vi "Framework Configuration 1.0 JSON Flatten.vi"(8 "error in (no error)":errorcluster, 11 "framework configuration 1.0":T2) -> (0 "error out":errorcluster, 2 "dsf version":T1, 3 "dsf configuration json":string)   [LabVIEW 2017, in "DSF Core.lvlib" / "Configuration Session.lvclass"]
uses:
  Configuration Session.lvclass
  Typedefs/DSF Version Info.ctl
  DSF Core.lvlib
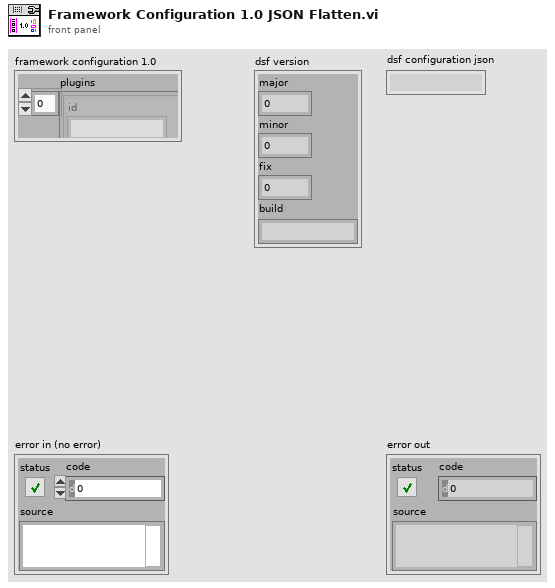
[diagram p1: front panel]
types:
  T1 = typedef "DSF Core.lvlib/DSF Version Info.ctl" = cluster{"major":u32, "minor":u32, "fix":u32, "build":string}
  T2 = cluster{"plugins":cluster{"id":string, "values":cluster{"components":string[], "timing":cluster{"priority":u64, "decimation":u64, "offset":u64}, "group ids":string[], "settings id":string, "threads":cluster{"buffer converter settings":cluster{"key":string, "value":string}[], "transceiver settings":cluster{"key":string, "value":string}[], "custom settings":cluster{"key":string, "value":string}[], "processor":i32, "priority offset":i16}[]}}[], "groups":cluster{"id":string, "values":cluster{"direction":i32, "timing":cluster{"priority":u64, "decimation":u64, "offset":u64}, "transfer ids":string[], "settings id":string, "thread":i32, "timeout behavior":u8}}[], "transfers":cluster{"id":string, "values":cluster{"byte order":i32, "channel ids":string[], "settings id":string}}[], "channels":cluster{"id":string, "values":cluster{"string buffer offset":u64, "string data type":i32, "engine data type":i32, "settings id":string, "units":string}}[], "settings":cluster{"id":string, "values":cluster{"key":string, "value":string}[]}[]}
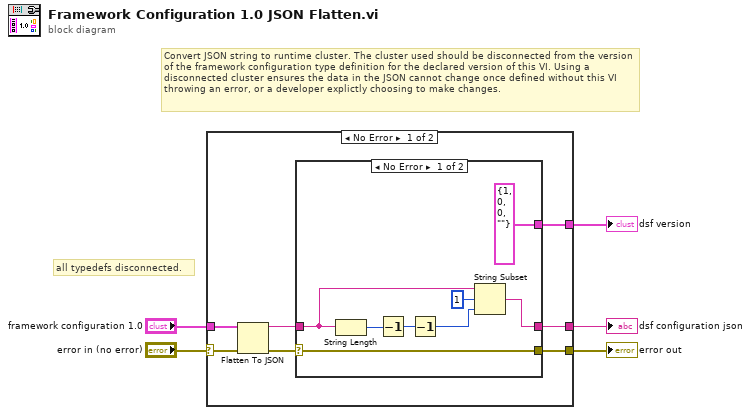
[diagram p0: block diagram]
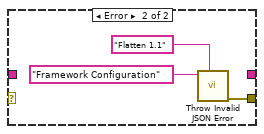
[diagram p2: hidden frame]
diagram:
  # "all typedefs disconnected."
  # "Convert JSON string to runtime cluster. The cluster used should be disconnected from the version of the framework configuration type definition for the declared version of this VI. Using a disconnected cluster ensures the data in the JSON cannot change once defined without this VI throwing an error, or a developer explictly choosing to make changes."
  n1 = case shown="No Error" "error in (no error)" {
    selector: "error in (no error)" -> [w9 w24]
    tunnel: [w11 w24] -> w5
    tunnel: "framework configuration 1.0" -> [w8 _]
    tunnel: [w7 _] -> w3
    tunnel: [w6 _] -> w1
    frame No Error {
      n2 = Flatten To JSON(anything=w8, error in (no error)=w9) -> (JSON string=w10:string, 11:w12:errorcluster)  [unwired: 1 in]
      n3 = case shown="No Error" w12 {
        selector: w12 -> [w20 _]
        tunnel: [w20 w23] -> w11
        tunnel: w10 -> [w18 _]
        tunnel: [w19 _] -> w7
        tunnel: [T1 {"major"=1, "minor"=0, "fix"=0, "build"=""} ("dsf version") _] -> w6
        frame No Error {
          n4 = String Length(string=w18) -> (length=w16:i32)
          n5 = Decrement(x=w16) -> (x-1=w15:i32)
          n6 = Decrement(x=w15) -> (x-1=w14:i32)
          n7 = String Subset(string=w18, offset (0)=1, length (rest)=w14) -> (substring=w19:string)
        }
        frame Error {
          n8 = call "Throw Invalid JSON Error.vi"("error source vi name"="Flatten 1.1", "name"="Framework Configuration") -> ("error out"=w23:errorcluster)  [unwired: 9 in]
        }
      }
    }
    frame Error {
    }
  }
  "dsf configuration json" <- w3
  "error out" <- w5
  "dsf version" <- w1
